vi "set_port.vi"(8 "error in (no error)":errorcluster, 10 "VISA resource name":refnum<visa-resource-name>, 11 "Motech-pps-1200 in":refnum<class "Motech-pps-1200.lvclass">) -> (0 "error in (no error) 2":errorcluster, 3 "Motech-pps-1200 out":refnum<class "Motech-pps-1200.lvclass">)   [LabVIEW 2017, in "Motech-pps-1200.lvclass"]
uses:
  Motech-pps-1200.lvclass
  DC_power_supply.lvclass
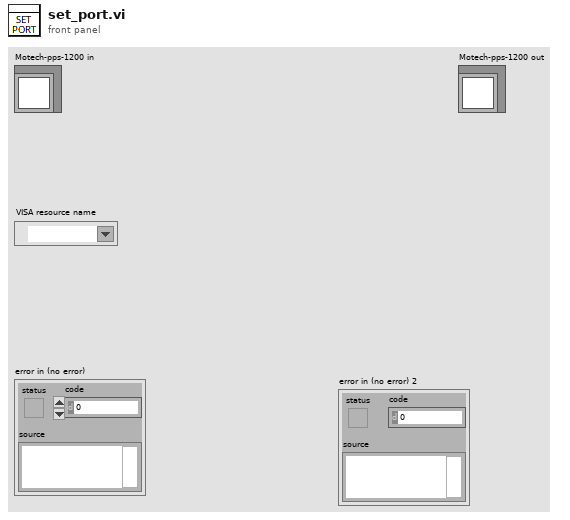
[diagram p1: front panel]
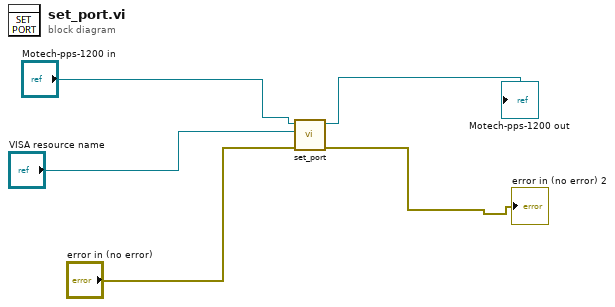
[diagram p0: block diagram]
diagram:
  n1 = call-parent "set_port.vi"("error in (no error)"="error in (no error)", "VISA resource name"="VISA resource name", "DC_power_supply in"="Motech-pps-1200 in") -> ("error out"=→"error in (no error) 2":errorcluster, "DC_power_supply out"=→"Motech-pps-1200 out":refnum<class "Motech-pps-1200.lvclass">)  [unwired: 7 in]
